vi "ZPL Transient ABORT.vi"(6 "Settle (1 mS)":u32=1, 8 "error":errorcluster, 11 "VISA":refnum<visa-resource-name>) -> (0 "error out":errorcluster, 3 "VISA out":refnum<visa-resource-name>)   [LabVIEW 2015]
doc: "This command cancels any trigger actions presently in process \n\nThis VI will wait for \"Settle\" milliseconds after setting the limit to allow the output to reach the new setting. If unwired, there will be no delay"
panel:
  # "Lambda ZPLUS \n Serial Port\n  DC Power Supplies"
  # "ABORT"
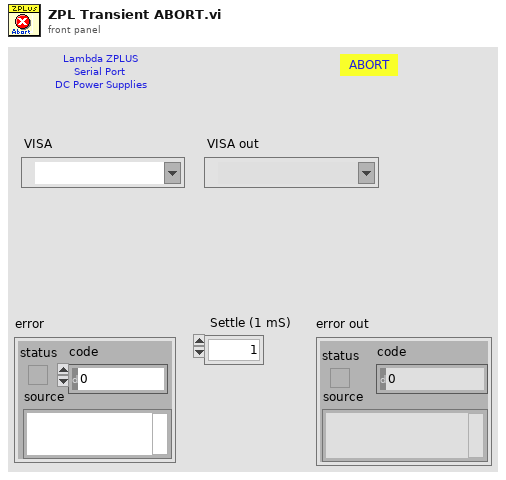
[diagram p1: front panel]
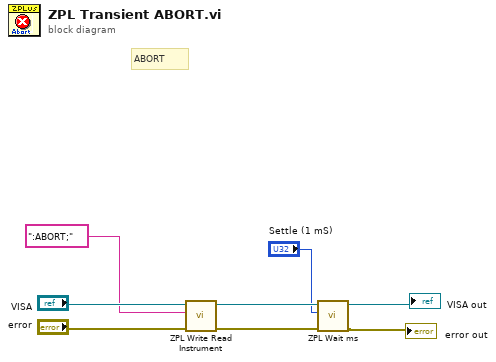
[diagram p0: block diagram]
diagram:
  # "ABORT"
  n1 = call "ZPL Write Read Instrument.vi"("error in"="error", "Write Command/Query SCPI"=":ABORT;", "VISA"="VISA") -> ("error out"=w5:errorcluster, "VISA  out"=w6:refnum<visa-resource-name>)  [unwired: 6 in, 1 out]
  n2 = call "ZPL Wait ms.vi"("error"=w5, "Delay (1 mS)"="Settle (1 mS)", "VISA"=w6) -> ("error out"=→"error out":errorcluster, "VISA out"=→"VISA out":refnum<visa-resource-name>)  [unwired: 7 in]
